vi "API Play Pause Background Music.vi"(8 "Error In":errorcluster, 11 "Function":enum16{"Pause", "Resume", "Next"}(ring)) -> (0 "error in (no error)":errorcluster)   [LabVIEW 2021, in "Sound Manager.lvlib"]
uses:
  Sound Manager.lvlib
  <vilib>/event_ctls.llb/usereventprio.ctl
  Architecture/Typedefs/Enum_Module_Name.ctl
  Architecture/Architecture.lvlib
  Architecture/Modules/Configuration/Configuration.lvlib
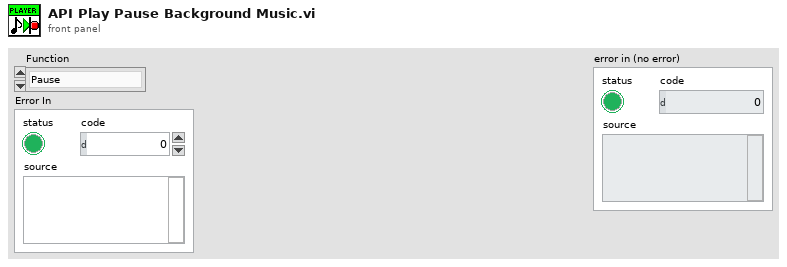
[diagram p1: front panel]
types:
  T1 = typedef "Configuration.lvlib/Enum_Module_Name.ctl" = enum16{"Configuration", "Error_Handler", "Log", "Database", "Controller", "UI Module", "Sound Manager"}
  T2 = typedef "usereventprio.ctl" = enum32{"high priority", "normal priority"}
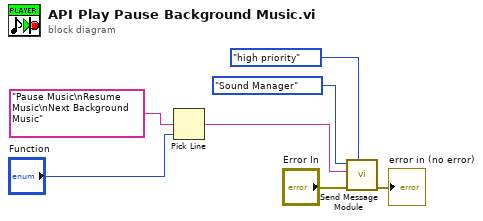
[diagram p0: block diagram]
diagram:
  n1 = Pick Line(multi-line string="Pause Music\nResume Music\nNext Background Music", line index="Function") -> (output string=w2:string)  [unwired: 1 in]
  n2 = call "Send Message Module.vi"("priority (normal)"=usereventprio."high priority", "Error In"="Error In", "Message"=w2, "Target ModuleName In"=Enum_Module_Name."Sound Manager") -> ("error in (no error)"=→"error in (no error)":errorcluster)  [unwired: 7 in]
